vi "NiFPGA Open.vi"(7 "Attribute":enum32{"Run (Default)", "No Run"}(ring), 8 "error in (no error)":errorcluster, 9 "Resource":string, 10 "Signature":string, 11 "Bitfile":string) -> (0 "error out":errorcluster, 2 "Status":i32, 3 "Session Out":u32)   [LabVIEW 2020, in "SEECD Engine.lvlib"]
doc: "Opens a session to the FPGA. This call ensures that the contents of the bitfile are programmed to the FPGA. The FPGA runs unless the NiFpga_OpenAttribute_NoRun attribute is used. Because different operating systems have different default current working directories for applications, you must pass an absolute path for the bitfile parameter. If you pass only the filename instead of an absolute path, the operating system may not be able to locate the bitfile. For example, the default current working directories are C:\\ni-rt\\system\\ for Phar Lap ETS and /c/ for VxWorks. Because the generated *_Bitfile constant is a #define to a string literal, you can use C/C++ string-literal concatenation to form an absolute path. For example, if the bitfile is in the root directory of a Phar Lap ETS system, pass the following for the bitfile parameter. \"C:\\\\\" NiFpga_MyApplication_Bitfile"
uses:
  SEECD Engine.lvlib
  NiFpga.dll
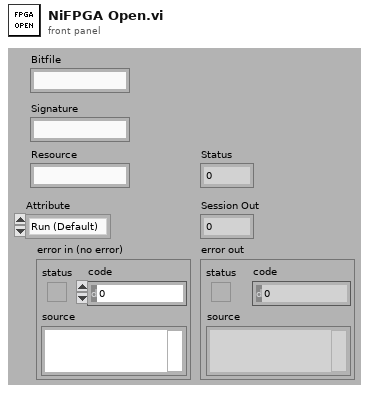
[diagram p1: front panel]
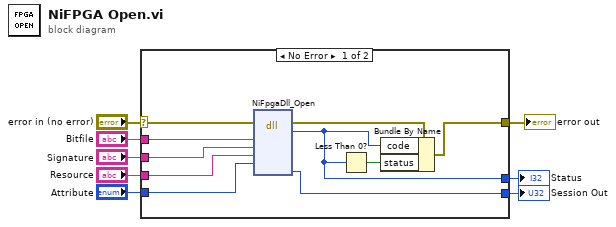
[diagram p0: block diagram]
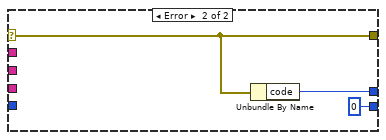
[diagram p2: hidden frame]
diagram:
  n1 = case shown="No Error" "error in (no error)" {
    selector: "error in (no error)" -> [w18 w21]
    tunnel: [w15 w21] -> w7
    tunnel: [w17 u32 0 ("Session")] -> w6
    tunnel: [w13 w20] -> w5
    tunnel: "Attribute" -> [w12 _]
    tunnel: "Resource" -> [w11 _]
    tunnel: "Signature" -> [w10 _]
    tunnel: "Bitfile" -> [w9 _]
    frame No Error {
      n2 = dll-call lib="NiFpga.dll" fn="NiFpgaDll_Open"(error in=w18, "Bitfile"=w9, "Signature"=w10, "Resource"=w11, "Attribute"=w12) -> (error out=w16:errorcluster, "Status"=w13:i32, "Session"=w17:u32)  [unwired: 7 in, 1 out]
      n3 = Less Than 0?(x=w13) -> (x < 0?=w14:bool)
      n4 = Bundle By Name(cluster=w16, "code"=w13, "status"=w14) -> (w15:errorcluster)
    }
    frame Error {
      n5 = Unbundle By Name(w21) -> ("code"=w20:i32)
    }
  }
  "error out" <- w7
  "Session Out" <- w6
  "Status" <- w5
